vi "testLoopbackUDP.vi"(8 "error in (no error)":errorcluster, 11 "TestCase in":refnum<class "DSF CD UDP System Tests.lvclass">) -> (0 "error out":errorcluster, 3 "TestCase out":refnum<class "DSF CD UDP System Tests.lvclass">)   [LabVIEW 2020, in "DSF CD UDP System Tests.lvclass"]
uses:
  DSF CD UDP System Tests.lvclass
  <vilib>/addons/_JKI Toolkits/VI Tester/TestCase.llb/TestCase.lvclass
  <vilib>/NI VeriStand/Execution/Workspace/NI_VS Workspace ExecutionAPI.lvlib
  b55b5565-dc34-4e51-bcfa-5a6cba25043e.vi
  df0c3853-f0b6-44a9-ad36-32614d313efc.vi
  <vilib>/NI/VeriStand Custom Device Testing Tools/VeriStandTestCase/VeriStandTestCase.lvclass
  <vilib>/NI VeriStand/Execution/Workspace/NI VeriStand - Set Single Channel Value.vi
  <vilib>/NI VeriStand/Execution/Workspace/NI VeriStand - Get Single Channel Value.vi
  C:/Program Files (x86)/National Instruments/LabVIEW 2020/vi.lib/NI/VeriStand Custom Device Testing Tools/VeriStandTestCase/VeriStandTestCase.lvclass
  C:/Program Files (x86)/National Instruments/LabVIEW 2020/vi.lib/addons/_JKI Toolkits/VI Tester/TestCase.llb/TestCase.lvclass
  C:/Users/nitest/Desktop/Git/niveristand-data-sharing-framework-custom-device/Source/Custom Device/Tests/System/UDP/DSF CD UDP System Tests.lvclass
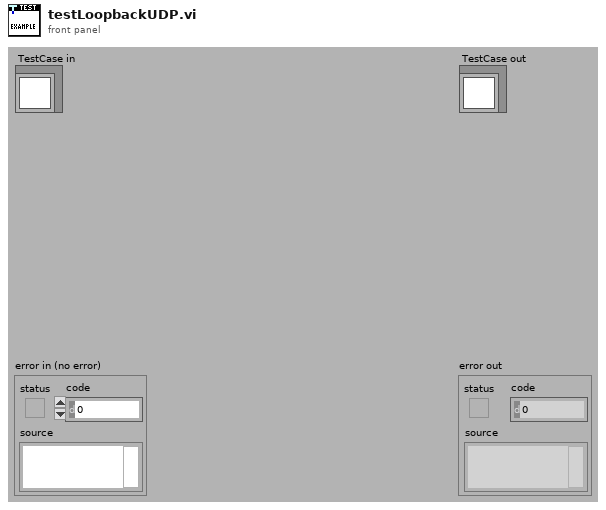
[diagram p1: front panel]
types:
  T1 = typedef "VeriStandTestUtilities.lvlib/TargetPlatform.ctl" = enum16{"Windows", "Linux64CRIO", "Linux64PXI", "LinuxARM", "PharLap"}
  T2 = typedef "NI_VS Workspace ExecutionAPI.lvlib/WorkspaceAPI.ctl" = refnum<k24>
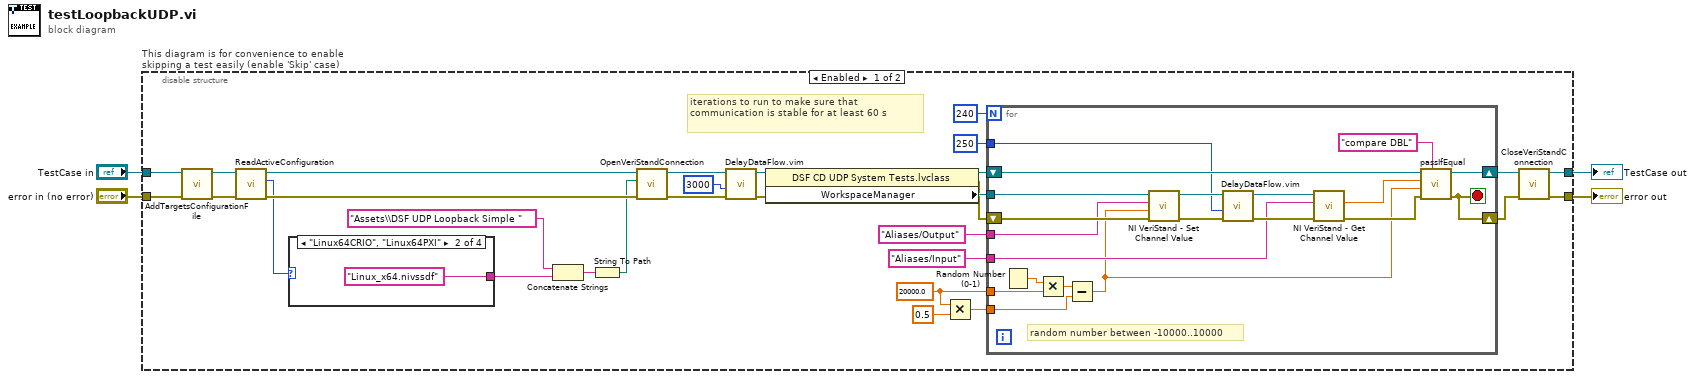
[diagram p0: block diagram]
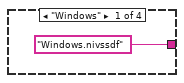
[diagram p2: hidden frame]
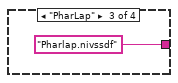
[diagram p3: hidden frame]
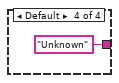
[diagram p4: hidden frame]
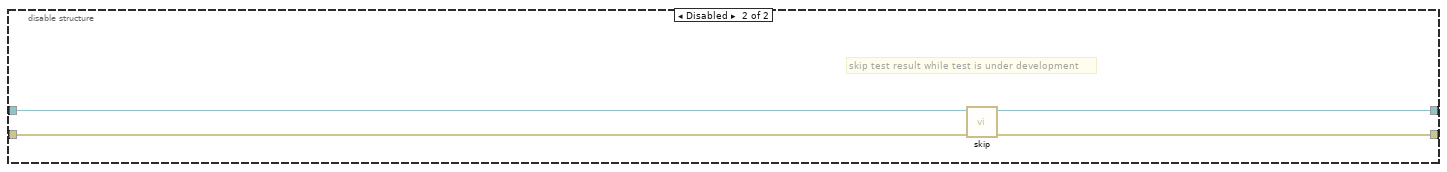
[diagram p5: hidden frame]
diagram:
  n1 = disable-structure "This diagram is for convenience to enable skipping a test easily (enable 'Skip' case)" shown="Enabled" {
    disable-tunnel: "TestCase in" -> [w12 w60]
    disable-tunnel: [w7 w58] -> w1
    disable-tunnel: [w5 w59] -> w2
    disable-tunnel: "error in (no error)" -> [w10 w57]
    frame Enabled {
      w21 = 20000.0 ("y")
      # "iterations to run to make sure that communication is stable for at least 60 s"
      n2 = call <vilib>:"AddTargetsConfigurationFile.vi"("error in (no error)"=w10, "VeriStandTestCase in"=w12) -> ("error out"=w9:errorcluster, "VeriStandTestCase out"=w11:refnum<class "DSF CD UDP System Tests.lvclass">)  [unwired: 8 in]
      n3 = call-dynamic "ReadActiveConfiguration.vi"("error in (no error)"=w9, "VeriStandTestCase in"=w11) -> ("error out"=w19:errorcluster, "Target Platform"=w17:T1, "VeriStandTestCase out"=w18:refnum<class "DSF CD UDP System Tests.lvclass">)  [unwired: 7 in]
      n4 = case shown="\"Linux64CRIO\", \"Linux64PXI\"" w17 {
        tunnel: ["Windows.nivssdf" ("Channel") "Linux_x64.nivssdf" ("Channel") "Pharlap.nivssdf" ("Channel") "Unknown" ("Channel")] -> w15
        frame "Windows" {
        }
        frame "Linux64CRIO", "Linux64PXI" {
        }
        frame "PharLap" {
        }
        frame Default {
        }
      }
      n5 = Concatenate Strings("Assets\\DSF UDP Loopback Simple " ("Channel"), w15) -> (w14:string)
      n6 = String To Path(string=w14) -> (path=w13:path)
      n7 = call-dynamic "OpenVeriStandConnection.vi"("error in (no error)"=w19, "System Definition File"=w13, "VeriStand Test Case in"=w18) -> ("error out"=w26:errorcluster, "VeriStand Test Case out"=w33:refnum<class "DSF CD UDP System Tests.lvclass">)  [unwired: 6 in, 1 out]
      n8 = call "DelayDataFlow.vim"("value in"=w26, "milliseconds to wait"=u32 3000) -> ("value out"=w25:errorcluster)  [unwired: 2 in, 1 out]
      n9 = property class="DSF CD UDP System Tests.lvclass"(reference=w33, error in=w25) -> (reference out=w28:refnum<class "DSF CD UDP System Tests.lvclass">, error out=w31:errorcluster, "WorkspaceManager"=w32:T2)
      n10 = Multiply(x=w21, y=0.5) -> (x*y=w22:dbl)
      n11 = for {
        N: 240 -> [_]
        tunnel: w32 -> [w56]
        tunnel: "Aliases/Input" ("Channel") -> [w51]
        tunnel: "Aliases/Output" ("Channel") -> [w50]
        shift-right: [w38] -> w6
        shift-left: w31 -> [w55]
        shift-right: [w46] -> w8
        shift-left: w28 -> [w47]
        tunnel: w22 -> [w41]
        tunnel: w21 -> [w40]
        tunnel: u32 250 ("milliseconds to wait") -> [w39]
        stop <- w38 stop-if-true
        # "random number between -10000..10000"
        n12 = Random Number (0-1)() -> (number: 0 to 1=w45:dbl)
        n13 = Multiply(x=w45, y=w40) -> (x*y=w44:dbl)
        n14 = Subtract(x=w44, y=w41) -> (x-y=w43:dbl)
        n15 = call-poly <vilib>:"NI VeriStand - Set Channel Value.vi"("error in (no error)"=w55, "Value"=w43, "Channel"=w50, "WorkspaceManager in"=w56) -> ("error out"=w54:errorcluster, "WorkspaceManager out"=w52:T2)  [unwired: 6 in]
        n16 = call "DelayDataFlow.vim"("value in"=w54, "milliseconds to wait"=w39) -> ("value out"=w53:errorcluster)  [unwired: 2 in, 1 out]
        n17 = call-poly <vilib>:"NI VeriStand - Get Channel Value.vi"("error in (no error)"=w53, "Channel"=w51, "WorkspaceManager in"=w52) -> ("error out"=w49:errorcluster, "Value"=w48:dbl)  [unwired: 6 in, 1 out]
        n18 = call-dynamic "passIfEqual.vi"("custom report message (\"\")"="compare DBL" ("custom report message (\"\")"), "error in (no error)"=w49, "y"=w43, "x"=w48, "TestCase in"=w47) -> ("error out"=w38:errorcluster, "TestCase out"=w46:refnum<class "DSF CD UDP System Tests.lvclass">)  [unwired: 5 in]
      }
      n19 = call-dynamic "CloseVeriStandConnection.vi"("error in (no error)"=w6, "VeriStand Test Case in"=w8) -> ("error out"=w5:errorcluster, "VeriStand Test Case out"=w7:refnum<class "DSF CD UDP System Tests.lvclass">)  [unwired: 8 in]
    }
    frame Disabled {
      # "skip test result while test is under development"
      n20 = call <vilib>:"skip.vi"("error in (no error)"=w57, "TestCase in"=w60) -> ("error out"=w59:errorcluster, "TestCase out"=w58:refnum<class "DSF CD UDP System Tests.lvclass">)  [unwired: 8 in]
    }
  }
  "error out" <- w2
  "TestCase out" <- w1
